vi "SplitUDPPacks.vi"(8 "pack size":i32=50, 11 "total size":i32) -> (3 "output array":i32[](array[numeric]))   [LabVIEW 2017, in "UDP++.lvlib"]
doc: "Calculates how to divide size bytes into packets of y bytes. The leading elements of output array are y and the last element carries the remainder, so size 201 with y 50 gives [50,50,50,50,1]."
uses:
  UDP++.lvlib
panel:
  out "floor(x/y)":i32
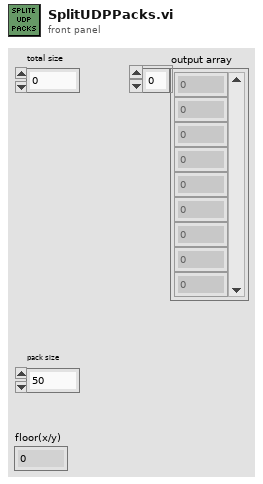
[diagram p1: front panel]
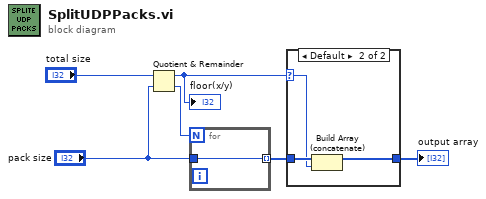
[diagram p0: block diagram]
diagram:
  n1 = Quotient & Remainder(x="total size", y="pack size") -> (x-y*floor(x/y)=w2:i32, floor(x/y)=w3:i32)
  "floor(x/y)" <- w2
  n2 = for {
    N: w3 -> [_]
    tunnel: "pack size" -> [w7]
    tunnel: [w7] -> w5 mode=indexing
  }
  n3 = case shown="Default" w2 {
    selector: w2 -> [_ w10]
    tunnel: w5 -> [w8 w11]
    tunnel: [w8 w9] -> w4
    frame 0 {
    }
    frame Default {
      n4 = Build Array (concatenate)(w11, w10) -> (w9:i32[])
    }
  }
  "output array" <- w4
